vi "pharosWriteDynReg.vi"(1 "triggers":u8[](array[numeric])) -> ()   [LabVIEW 2017]
uses:
  <vilib>/DAQmx/write.llb/DAQmx Write (Digital 1D U8 1Chan NSamp).vi
  globalDevices.vi
  <vilib>/DAQmx/miscellaneous.llb/DAQmx Fill In Error Info.vi
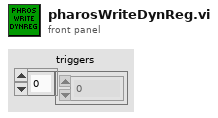
[diagram p1: front panel]
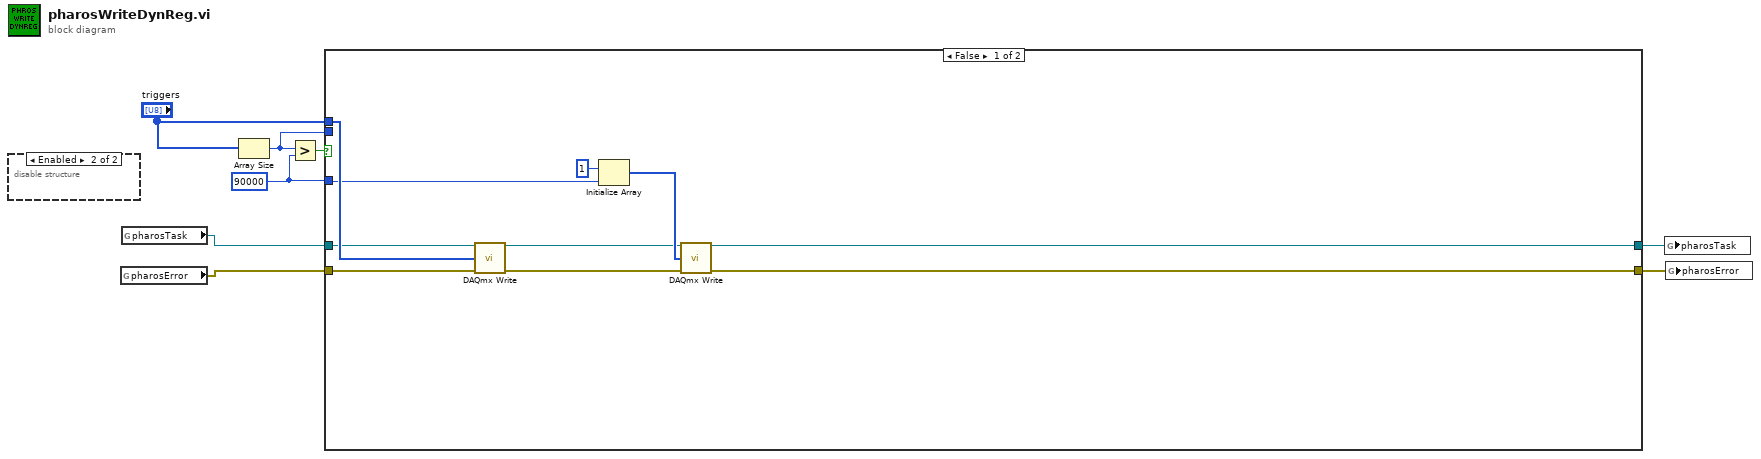
[diagram p0: block diagram]
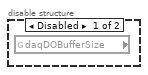
[diagram p2: hidden frame]
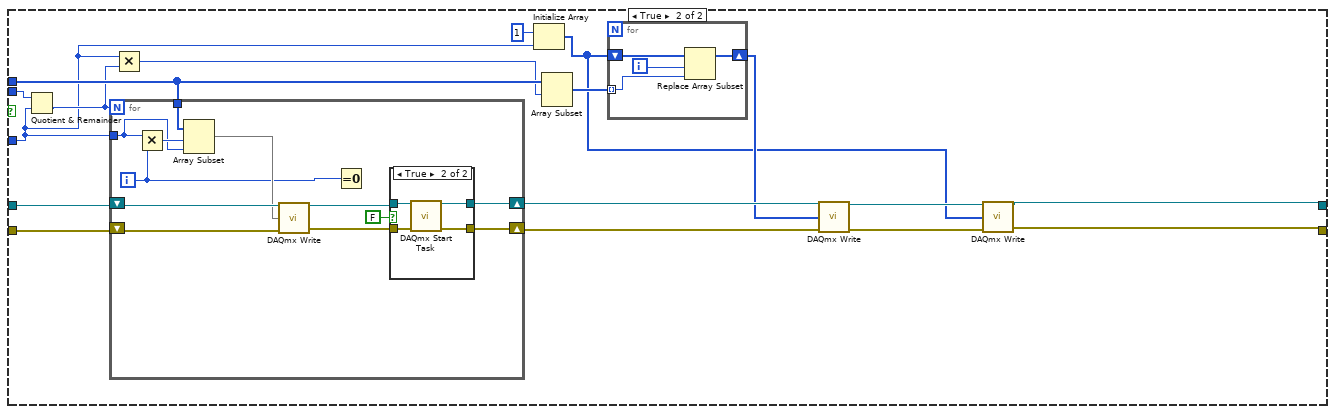
[diagram p3: hidden frame]
diagram:
  w1 = 90000
  n1 = disable-structure shown="Enabled" {
    frame Disabled {
      n2 = global read "globalDevices.vi" "daqDOBufferSize"() -> ()  [unwired: 1 out]
    }
    frame Enabled {
    }
  }
  n3 = global read "globalDevices.vi" "pharosError"() -> (w5:errorcluster)
  n4 = global read "globalDevices.vi" "pharosTask"() -> (w6:refnum<k21>)
  n5 = Array Size(array="triggers") -> (size(s)=w4:i32)
  n6 = Greater?(x=w4, y=w1) -> (0:w8:bool)
  n7 = case shown="False" w8 {
    tunnel: "triggers" -> [w18 w31]
    tunnel: w6 -> [w17 w34]
    tunnel: w5 -> [w16 w33]
    tunnel: [w10 w21] -> w3
    tunnel: [w11 w20] -> w2
    tunnel: w4 -> [_ w35]
    tunnel: w1 -> [w9 w25]
    frame False {
      n8 = call-poly <vilib>:"DAQmx Write.vi"("task/channels in"=w17, "data"=w18, "error in"=w16) -> ("task out"=w13:refnum<k21>, "error out"=w12:errorcluster)  [unwired: 10 in, 1 out]
      n9 = Initialize Array(u8 1 ("element"), w9) -> (w14:u8[])
      n10 = call-poly <vilib>:"DAQmx Write.vi"("task/channels in"=w13, "data"=w14, "error in"=w12) -> ("task out"=w10:refnum<k21>, "error out"=w11:errorcluster)  [unwired: 10 in, 1 out]
    }
    frame True {
      n11 = Quotient & Remainder(x=w35, y=w25) -> (floor(x/y)=w26:i32)  [unwired: 1 out]
      n12 = for {
        N: w26 -> [_]
        tunnel: w31 -> [w51]
        tunnel: w25 -> [w42]
        shift-right: [w44] -> w29
        shift-left: w34 -> [w49]
        shift-right: [w43] -> w28
        shift-left: w33 -> [w48]
        i -> [w41]
        n13 = Multiply(x=w42, y=w41) -> (x*y=w50:i32)
        n14 = Array Subset(array=w51, index=w50, length=w42) -> (w47:u8[])
        n15 = call-poly <vilib>:"DAQmx Write.vi"("task/channels in"=w49, "data"=w47, "error in"=w48) -> ("task out"=w46:refnum<k21>, "error out"=w45:errorcluster)  [unwired: 10 in, 1 out]
        n16 = Equal To 0?(x=w41) -> ()  [unwired: 1 out]
        n17 = case shown="True" FALSE {
          tunnel: w45 -> [w52 w57]
          tunnel: w46 -> [w53 w56]
          tunnel: [w52 w55] -> w43
          tunnel: [w53 w54] -> w44
          frame False {
          }
          frame True {
            n18 = call <vilib>:"DAQmx Start Task.vi"("task/channels in"=w56, "error in"=w57) -> ("task out"=w54:refnum<k21>, "error out"=w55:errorcluster)  [unwired: 12 in]
          }
        }
      }
      n19 = Multiply(x=w25, y=w26) -> (x*y=w24:i32)
      n20 = Initialize Array(u8 1 ("element"), w25) -> (w19:u8[])
      n21 = Array Subset(array=w31, index=w24) -> (w30:u8[])  [unwired: 1 in]
      n22 = for {
        tunnel: w30 -> [w37] mode=indexing
        shift-right: [w36] -> w27
        shift-left: w19 -> [w39]
        i -> [w38]
        n23 = Replace Array Subset(array=w39, new element=w37, index=w38) -> (w36:u8[])
      }
      n24 = call-poly <vilib>:"DAQmx Write.vi"("task/channels in"=w29, "data"=w27, "error in"=w28) -> ("task out"=w23:refnum<k21>, "error out"=w22:errorcluster)  [unwired: 10 in, 1 out]
      n25 = call-poly <vilib>:"DAQmx Write.vi"("task/channels in"=w23, "data"=w19, "error in"=w22) -> ("task out"=w21:refnum<k21>, "error out"=w20:errorcluster)  [unwired: 10 in, 1 out]
    }
  }
  n26 = global write "globalDevices.vi" "pharosTask"(w3) -> ()
  n27 = global write "globalDevices.vi" "pharosError"(w2) -> ()
